vi "PCA9535 - 0x22.vi"(8 "error in (no error)":errorcluster, 11 "handle":u64 format="%x") -> (0 "error out":errorcluster, 2 "0X22 Pass or Fail":bool, 3 "handle 2":u64)   [LabVIEW 2024]
panel:
  out "sizeTransferred (Output) 3":u32
  out "sizeTransferred (Output) 2":u32
  out "sizeTransferred (Output)":u32
  out "p/f1":bool
  out "p/f2":bool
  out "p/f3":bool
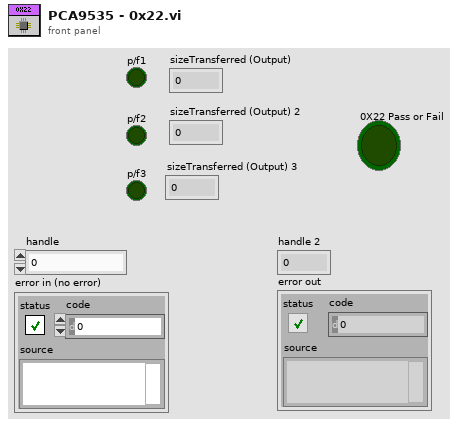
[diagram p1: front panel]
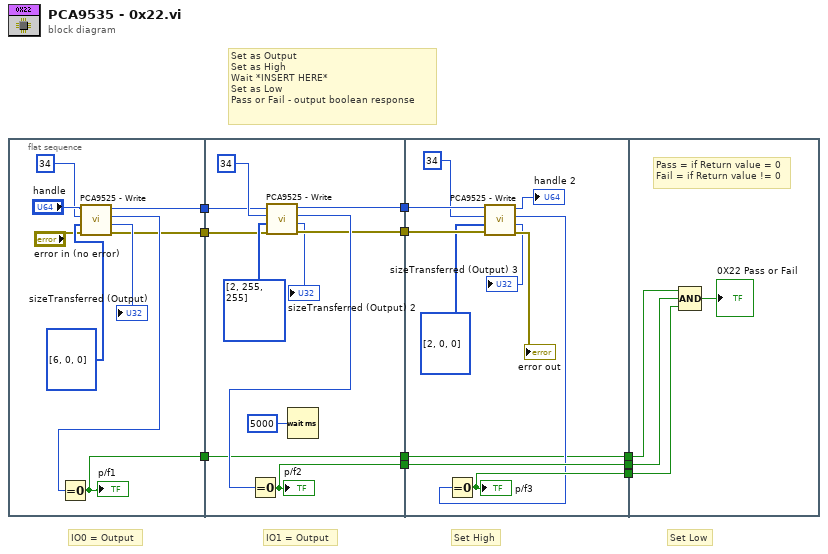
[diagram p0: block diagram]
diagram:
  # "Set Low"
  # "Set High"
  # "IO1 = Output"
  # "IO0 = Output"
  # "Set as Output \nSet as High\nWait *INSERT HERE*\nSet as Low\nPass or Fail - output boolean response"
  n1 = flat-sequence {
    tunnel: [w13] -> w3
    tunnel: [w12] -> w2
    tunnel: [w11] -> w1
    tunnel: [w29] -> w9
    tunnel: [w27] -> w7
    tunnel: [w26] -> w6
    tunnel: [w22] -> w4
    tunnel: w3 -> [w22]
    tunnel: w2 -> [w21]
    tunnel: w1 -> [w20]
    tunnel: [w41] -> w10
    tunnel: w9 -> [w40]
    tunnel: [w40] -> w8
    tunnel: w7 -> [w39]
    tunnel: w6 -> [w35]
    tunnel: [w31] -> w5
    tunnel: w4 -> [w31]
    tunnel: w10 -> [w45]
    tunnel: w8 -> [w43]
    tunnel: w5 -> [w42]
    frame #0 {
      n2 = call "PCA9525 - Write.vi"("error in (no error)"="error in (no error)", "buffer"=u8[] [6, 0, 0], "deviceAddress"=u8 34, "handle"="handle") -> ("error out"=w11:errorcluster, "sizeTransferred (Output)"=→"sizeTransferred (Output)":u32, "return (Output)"=w19:u64, "handle 2"=w12:u64)  [unwired: 4 in]
      n3 = Equal To 0?(x=w19) -> (x = 0?=w13:bool)
      "p/f1" <- w13
    }
    frame #1 {
      n4 = call "PCA9525 - Write.vi"("error in (no error)"=w20, "buffer"=u8[] [2, 255, 255], "deviceAddress"=u8 34, "handle"=w21) -> ("error out"=w26:errorcluster, "sizeTransferred (Output)"=→"sizeTransferred (Output) 2":u32, "return (Output)"=w28:u64, "handle 2"=w27:u64)  [unwired: 4 in]
      n5 = Equal To 0?(x=w28) -> (x = 0?=w29:bool)
      "p/f2" <- w29
      n6 = Wait (ms)(milliseconds to wait=u32 5000) -> ()  [unwired: 1 out]
    }
    frame #2 {
      n7 = call "PCA9525 - Write.vi"("error in (no error)"=w35, "buffer"=u8[] [2, 0, 0], "deviceAddress"=u8 34, "handle"=w39) -> ("error out"=→"error out":errorcluster, "sizeTransferred (Output)"=→"sizeTransferred (Output) 3":u32, "return (Output)"=w36:u64, "handle 2"=→"handle 2":u64)  [unwired: 4 in]
      n8 = Equal To 0?(x=w36) -> (x = 0?=w41:bool)
      "p/f3" <- w41
    }
    frame #3 {
      # "Pass = if Return value = 0\nFail = if Return value != 0"
      n9 = Compound Arithmetic op=AND(w42, w43, w45) -> (→"0X22 Pass or Fail":bool)
    }
  }
